vi "GuessPathFromName.vi"(4 "Don'tAppendName":bool, 6 "FolderSuffix":string, 7 "NewName":string, 9 "OldName":string, 10 "Stereo Type":T1(ring), 11 "PathIn":path) -> (3 "File Path":path)   [LabVIEW 2020, in "AbstractNode.lvclass"]
uses:
  <resource>/Framework/Providers/Open_GDS/UML/AbstractNode_class/AbstractNode.lvclass
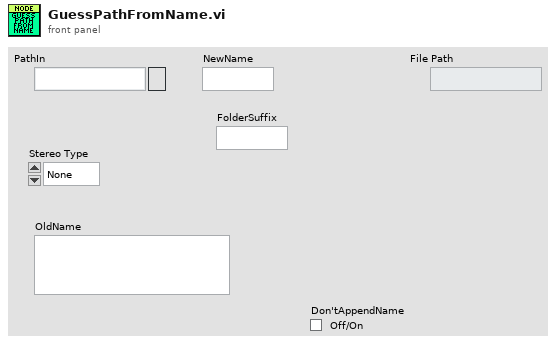
[diagram p1: front panel]
types:
  T1 = enum16{"None", "TYPE", "ENUM", "ABSTRACT", "ACTOR", "GUI", "SINGLETON", "SIGNAL", "BOUNDARY", "ENTITY", "CONTROL", "LEGACY", "APPLICATION", "VI", "LVLIB"}
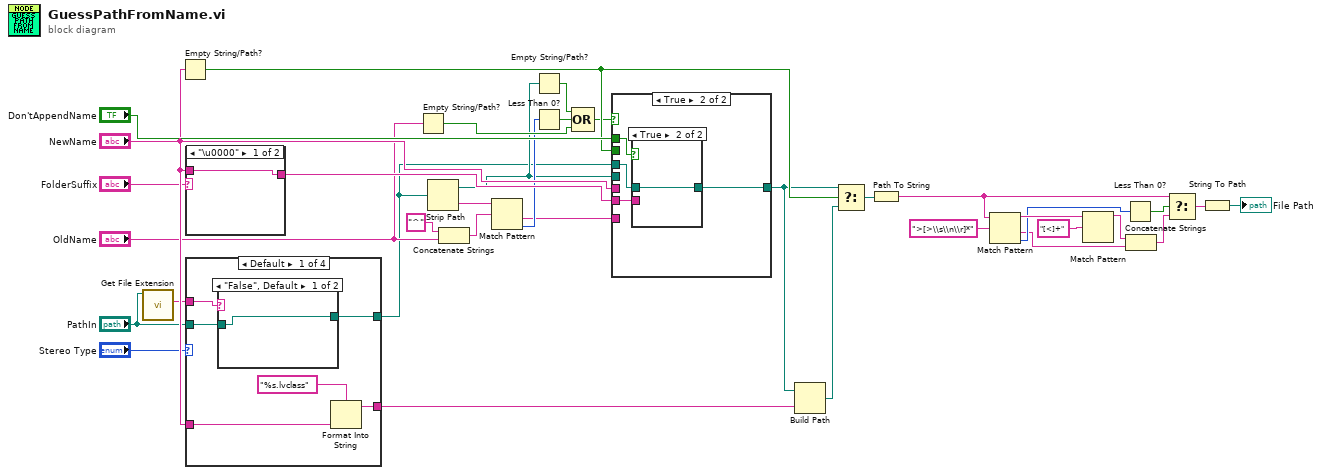
[diagram p0: block diagram]
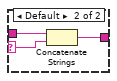
[diagram p2: hidden frame]
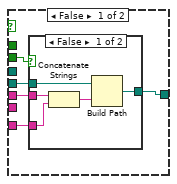
[diagram p3: hidden frame]
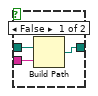
[diagram p5: hidden frame]
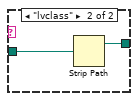
[diagram p6: hidden frame]
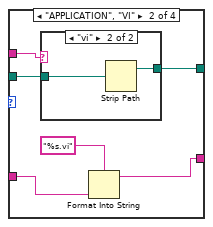
[diagram p7: hidden frame]
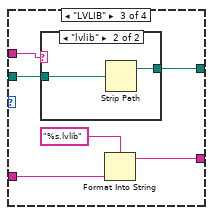
[diagram p9: hidden frame]
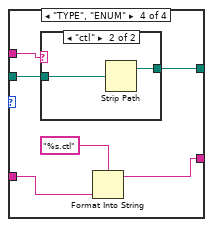
[diagram p11: hidden frame]
diagram:
  n1 = call <vilib>:"Get File Extension.vi"("file"="PathIn") -> ("lowercase file extension"=w3:string)  [unwired: 1 in, 9 out]
  n2 = Empty String/Path?(string/path="NewName") -> (empty?=w34:bool)
  n3 = case shown="\"\"" "FolderSuffix" {
    selector: "FolderSuffix" -> [_ w37]
    tunnel: "NewName" -> [w36 w39]
    tunnel: [w36 w38] -> w33
    frame "\u0000" {
    }
    frame Default {
      n4 = Concatenate Strings(w39, w37) -> (w38:string)
    }
  }
  n5 = case shown="Default" "Stereo Type" {
    tunnel: "PathIn" -> [w44 w53 w62 w71]
    tunnel: w3 -> [w45 w54 w63 w72]
    tunnel: "NewName" -> [w42 w51 w60 w69]
    tunnel: [w41 w50 w59 w68] -> w10
    tunnel: [w40 w49 w58 w67] -> w12
    frame Default {
      n6 = case shown="\"False\", Default" w45 {
        tunnel: w44 -> [w46 w48]
        tunnel: [w46 w47] -> w41
        frame "False", Default {
        }
        frame "lvclass" {
          n7 = Strip Path(path=w48) -> (stripped path=w47:path)  [unwired: 1 out]
        }
      }
      n8 = Format Into String(format string="%s.lvclass", w42) -> (resulting string=w40:string)  [unwired: 2 in, 1 out]
    }
    frame "APPLICATION", "VI" {
      n9 = case shown="\"vi\"" w54 {
        tunnel: w53 -> [w55 w57]
        tunnel: [w55 w56] -> w50
        frame "False", Default {
        }
        frame "vi" {
          n10 = Strip Path(path=w57) -> (stripped path=w56:path)  [unwired: 1 out]
        }
      }
      n11 = Format Into String(format string="%s.vi", w51) -> (resulting string=w49:string)  [unwired: 2 in, 1 out]
    }
    frame "LVLIB" {
      n12 = case shown="\"lvlib\"" w63 {
        tunnel: w62 -> [w64 w66]
        tunnel: [w64 w65] -> w59
        frame "False", Default {
        }
        frame "lvlib" {
          n13 = Strip Path(path=w66) -> (stripped path=w65:path)  [unwired: 1 out]
        }
      }
      n14 = Format Into String(format string="%s.lvlib", w60) -> (resulting string=w58:string)  [unwired: 2 in, 1 out]
    }
    frame "TYPE", "ENUM" {
      n15 = case shown="\"ctl\"" w72 {
        tunnel: w71 -> [w73 w75]
        tunnel: [w73 w74] -> w68
        frame "False", Default {
        }
        frame "ctl" {
          n16 = Strip Path(path=w75) -> (stripped path=w74:path)  [unwired: 1 out]
        }
      }
      n17 = Format Into String(format string="%s.ctl", w69) -> (resulting string=w67:string)  [unwired: 2 in, 1 out]
    }
  }
  n18 = Empty String/Path?(string/path="OldName") -> (empty?=w18:bool)
  n19 = Strip Path(path=w10) -> (stripped path=w13:path, name=w6:string)
  n20 = Concatenate Strings("^" ("string"), "OldName") -> (w8:string)
  n21 = Match Pattern(string=w6, regular expression=w8) -> (after substring=w9:string, offset past match=w15:i32)  [unwired: 3 out]
  n22 = Empty String/Path?(string/path=w13) -> (empty?=w16:bool)
  n23 = Less Than 0?(x=w15) -> (x < 0?=w17:bool)
  n24 = Compound Arithmetic op=OR(w16, w17, w18) -> (w19:bool)
  n25 = case shown="True" w19 {
    tunnel: w10 -> [_ w90]
    tunnel: [w79 w89] -> w11
    tunnel: w13 -> [w80 _]
    tunnel: "NewName" -> [w78 _]
    tunnel: w9 -> [w77 _]
    tunnel: w33 -> [_ w88]
    tunnel: w34 -> [w76 _]
    tunnel: "Don'tAppendName" -> [_ w87]
    frame False {
      n26 = case shown="False" w76 {
        tunnel: w80 -> [w85 w86]
        tunnel: [w84 w86] -> w79
        tunnel: w78 -> [w83 _]
        tunnel: w77 -> [w82 _]
        frame False {
          n27 = Concatenate Strings(w83, w82) -> (w81:string)
          n28 = Build Path(base path=w85, name or relative path=w81) -> (appended path=w84:path)
        }
        frame True {
        }
      }
    }
    frame True {
      n29 = case shown="True" w87 {
        tunnel: w90 -> [w93 w94]
        tunnel: [w92 w94] -> w89
        tunnel: w88 -> [w91 _]
        frame False {
          n30 = Build Path(base path=w93, name or relative path=w91) -> (appended path=w92:path)
        }
        frame True {
        }
      }
    }
  }
  n31 = Build Path(base path=w11, name or relative path=w12) -> (appended path=w5:path)
  n32 = Select(t=w11, s=w34, f=w5) -> (s? t:f=w30:path)
  n33 = Path To String(path=w30) -> (string=w20:string)
  n34 = Match Pattern(string=w20, regular expression=">[>\\s\\n\\r]*") -> (before substring=w28:string, after substring=w23:string, offset past match=w25:i32)  [unwired: 2 out]
  n35 = Match Pattern(string=w28, regular expression="[<]+") -> (before substring=w24:string)  [unwired: 4 out]
  n36 = Less Than 0?(x=w25) -> (x < 0?=w26:bool)
  n37 = Concatenate Strings(w24, w23) -> (w22:string)
  n38 = Select(t=w20, s=w26, f=w22) -> (s? t:f=w21:string)
  n39 = String To Path(string=w21) -> (path=→"File Path":path)
